vi "Energy (1 Channel).vi"(7 "reset? (F)":bool, 8 "error in (no error)":errorcluster, 9 "start timestamp":timestamp, 10 "interval length [s]":dbl=0.2, 11 "power value":T2) -> (0 "error out":errorcluster, 1 "measurement timestamps":T1, 3 "energy value":T3)   [LabVIEW 2014, in "NI_EP_Basic.lvlib"]
doc: "Calculates the energy value from the power value for a specified interval. This VI returns the value of active energy, apparent energy, and reactive energy. Wire data to the <B>power value</B> input to determine the polymorphic instance to use or manually select the instance."
uses:
  <vilib>/addons/Electrical Power/Basic/NI_EP_Basic.lvlib
  <vilib>/addons/Electrical Power/Basic/Measurement/subVIs/basic_Energy Value.ctl
  <vilib>/addons/Electrical Power/Basic/Measurement/subVIs/basic_Power Value.ctl
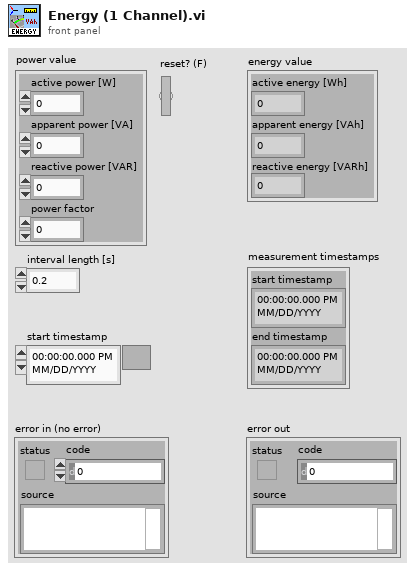
[diagram p1: front panel]
types:
  T1 = cluster{"start timestamp":timestamp, "end timestamp":timestamp}
  T2 = typedef "NI_EP_Basic.lvlib/basic_Power Value.ctl" = cluster{"active power [W]":dbl, "apparent power [VA]":dbl, "reactive power [VAR]":dbl, "power factor":dbl}
  T3 = typedef "NI_EP_Basic.lvlib/basic_Energy Value.ctl" = cluster{"active energy [Wh]":dbl, "apparent energy [VAh]":dbl, "reactive energy [VARh]":dbl}
  T4 = cluster{"start time stamp":timestamp, "end time stamp":timestamp}
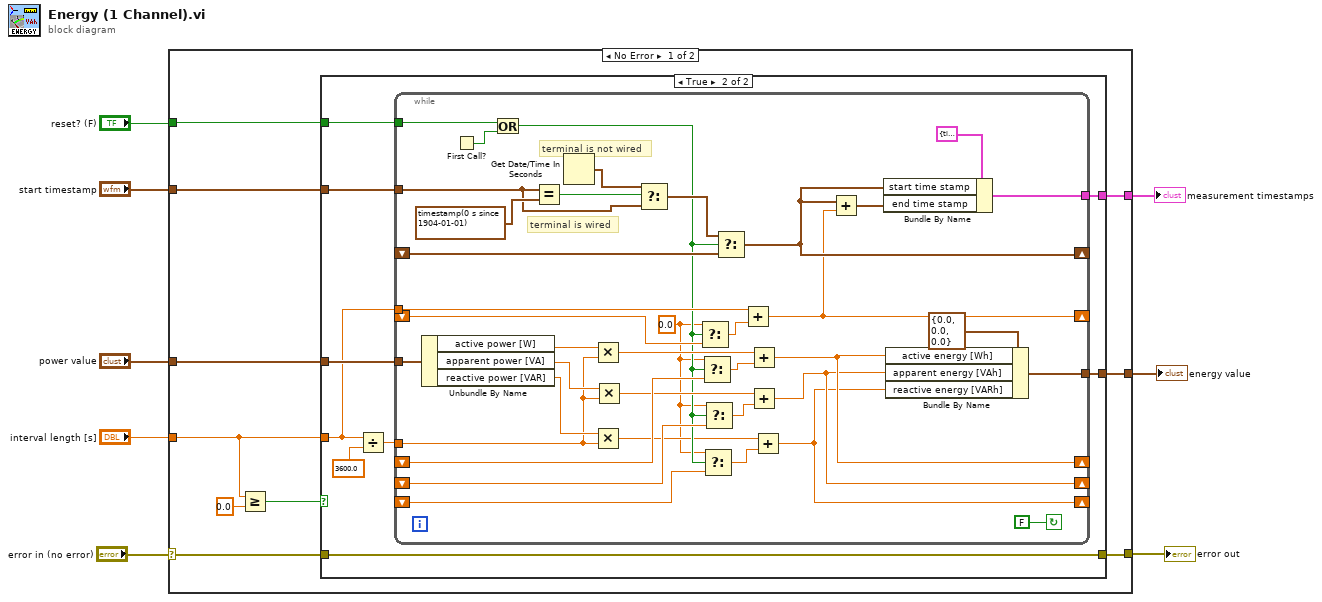
[diagram p0: block diagram]
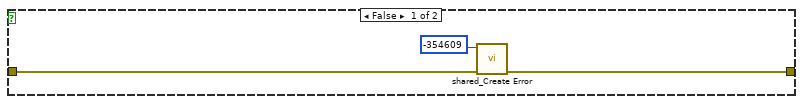
[diagram p2: hidden frame]
diagram:
  n1 = case shown="No Error" "error in (no error)" {
    selector: "error in (no error)" -> [w10 w69]
    tunnel: "power value" -> [w18 _]
    tunnel: "reset? (F)" -> [w17 _]
    tunnel: "start timestamp" -> [w16 _]
    tunnel: [w15 _] -> w5
    tunnel: [w14 _] -> w4
    tunnel: "interval length [s]" -> [w12 _]
    tunnel: [w9 w69] -> w1
    frame No Error {
      n2 = Greater Or Equal?(x=w12, y=0.0) -> (x >= y?=w11:bool)
      n3 = case shown="True" w11 {
        tunnel: w18 -> [_ w30]
        tunnel: w17 -> [_ w28]
        tunnel: w16 -> [_ w27]
        tunnel: [_ w26] -> w15
        tunnel: [_ w25] -> w14
        tunnel: w12 -> [_ w23]
        tunnel: w10 -> [w20 w22]
        tunnel: [w19 w22] -> w9
        frame False {
          n4 = call <vilib>:"shared_Create Error.vi"("error in (no error)"=w20, "error code (0)"=-354609) -> ("error out"=w19:errorcluster)  [unwired: 9 in]
        }
        frame True {
          n5 = Divide(x=w23, y=3600.0) -> (x/y=w24:dbl)
          n6 = while {
            tunnel: w30 -> [w68]
            tunnel: w28 -> [w66]
            tunnel: w27 -> [w62]
            tunnel: w24 -> [w50]
            tunnel: [w58] -> w26
            tunnel: [w56] -> w25
            shift-right: [w32] -> _
            shift-left: _ -> [w33]
            shift-right: [w37] -> _
            shift-left: _ -> [w40]
            shift-right: [w43] -> _
            shift-left: _ -> [w44]
            shift-right: [w47] -> _
            shift-left: _ -> [w48]
            shift-right: [w52] -> _
            shift-left: _ -> [w51]
            tunnel: w23 -> [w46]
            stop <- FALSE continue-if-true
            w31 = 0.0 ("t")
            # "terminal is wired"
            # "terminal is not wired"
            n7 = Unbundle By Name(w68) -> ("active power [W]"=w61:dbl, "apparent power [VA]"=w53:dbl, "reactive power [VAR]"=w60:dbl)
            n8 = First Call?() -> (First Call?: T/F=w67:bool)
            n9 = Or(x=w66, y=w67) -> (x .or. y?=w35:bool)
            n10 = Equal?(x=w62, y=timestamp(0 s since 1904-01-01) ("time stamp")) -> (x = y?=w63:bool)
            n11 = Get Date/Time In Seconds() -> (seconds since 1Jan1904=w65:timestamp)
            n12 = Multiply(x=w61, y=w50) -> (x*y=w42:dbl)
            n13 = Multiply(x=w60, y=w50) -> (x*y=w34:dbl)
            n14 = Multiply(x=w53, y=w50) -> (x*y=w38:dbl)
            n15 = Select(t=w65, s=w63, f=w62) -> (s? t:f=w54:timestamp)
            n16 = Select(t=w31, s=w35, f=w48) -> (s? t:f=w45:dbl)
            n17 = Select(t=w31, s=w35, f=w44) -> (s? t:f=w41:dbl)
            n18 = Select(t=w31, s=w35, f=w33) -> (s? t:f=w36:dbl)
            n19 = Select(t=w31, s=w35, f=w40) -> (s? t:f=w39:dbl)
            n20 = Select(t=w54, s=w35, f=w51) -> (s? t:f=w52:timestamp)
            n21 = Add(x=w46, y=w45) -> (x+y=w47:dbl)
            n22 = Add(x=w42, y=w41) -> (x+y=w43:dbl)
            n23 = Add(x=w38, y=w39) -> (x+y=w37:dbl)
            n24 = Add(x=w34, y=w36) -> (x+y=w32:dbl)
            n25 = Add(x=w52, y=w47) -> (x+y=w49:timestamp)
            n26 = Bundle By Name(cluster=T4 {"start time stamp"=timestamp(0 s since 1904-01-01), "end time stamp"=timestamp(0 s since 1904-01-01)} ("measurement time stamps"), "start time stamp"=w52, "end time stamp"=w49) -> (w58:T4)
            n27 = Bundle By Name(cluster=T3 {"active energy [Wh]"=0.0, "apparent energy [VAh]"=0.0, "reactive energy [VARh]"=0.0} ("energy  value"), "active energy [Wh]"=w43, "apparent energy [VAh]"=w37, "reactive energy [VARh]"=w32) -> (w56:T3)
          }
        }
      }
    }
    frame Error {
    }
  }
  "measurement timestamps" <- w5
  "energy value" <- w4
  "error out" <- w1
